vi "Reposition Index (SubVI).vi"(7 "Outer Bound":u16, 11 "Index":i16) -> (3 "Repositioned Index":i16)   [LabVIEW 2015]
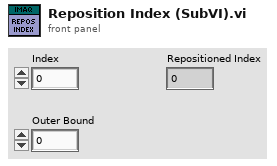
[diagram p1: front panel]
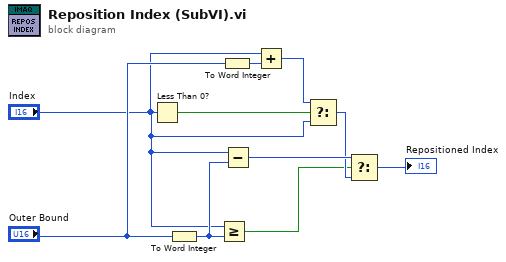
[diagram p0: block diagram]
diagram:
  n1 = Less Than 0?(x="Index") -> (x < 0?=w2:bool)
  n2 = To Word Integer(number="Outer Bound") -> (16bit integer=w6:i16)
  n3 = Greater Or Equal?(x="Index", y=w6) -> (x >= y?=w5:bool)
  n4 = To Word Integer(number="Outer Bound") -> (16bit integer=w3:i16)
  n5 = Subtract(x="Index", y=w6) -> (x-y=w8:i16)
  n6 = Add(x="Index", y=w3) -> (x+y=w4:i16)
  n7 = Select(t=w4, s=w2, f="Index") -> (s? t:f=w7:i16)
  n8 = Select(t=w8, s=w5, f=w7) -> (s? t:f=→"Repositioned Index":i16)
